vi "PXIe-5172_Init.vi"(8 "Error In":errorcluster, 11 "Object in":refnum<class "PXIe-5172.lvclass">) -> (0 "Error Out":errorcluster, 3 "object out":refnum<class "PXIe-5172.lvclass">)   [LabVIEW 2023, in "HAL.lvlib" / "PXIe-5172.lvlib" / "PXIe-5172.lvclass"]
uses:
  PXIe-5172.lvclass
  PXIe-5172.lvclass/PXIe-5172.ctl
  Hardware_class/Hardware.lvclass
  D:/git/HAL/Hardware_class/Hardware.lvclass
  D:/git/HAL/PXIe-5172_class/PXIe-5172.lvclass
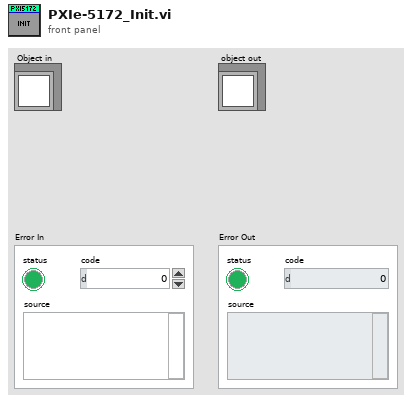
[diagram p1: front panel]
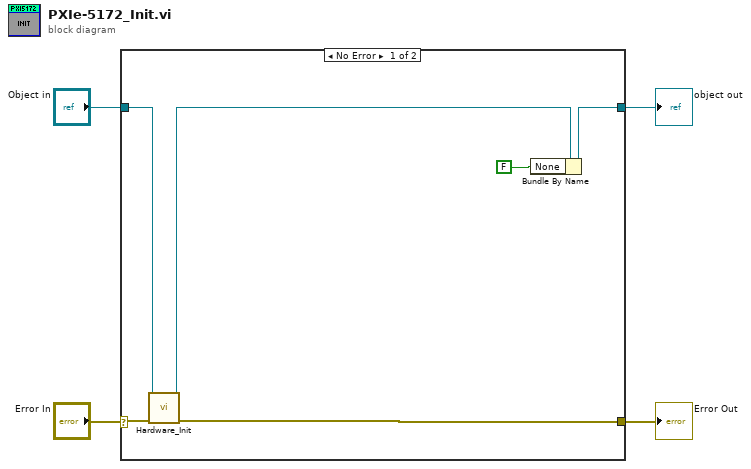
[diagram p0: block diagram]
diagram:
  n1 = case shown="No Error" "Error In" {
    selector: "Error In" -> [w8 w11]
    tunnel: [w10 w12] -> w4
    tunnel: "Object in" -> [w6 w12]
    tunnel: [w7 w11] -> w1
    frame No Error {
      n2 = call "Hardware_Init.vi"("Error In"=w8, "object in"=w6) -> ("Error Out"=w7:errorcluster, "object in"=w5:refnum<class "PXIe-5172.lvclass">)  [unwired: 8 in]
      n3 = Bundle By Name(cluster=w5, "None"=FALSE) -> (w10:refnum<class "PXIe-5172.lvclass">)
    }
    frame Error {
    }
  }
  "object out" <- w4
  "Error Out" <- w1
